vi "derivative.vi"(10 "Starting value":dbl, 11 "x":dbl) -> (3 "dx/dt":dbl)   [LabVIEW 2015]
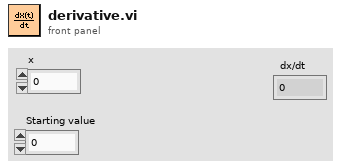
[diagram p1: front panel]
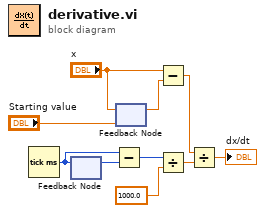
[diagram p0: block diagram]
diagram:
  n1 = Tick Count (ms)() -> (millisecond timer value=w5:u32)
  n2 = feedback #1() -> (w6:u32)  [unwired: 1 in]
  n3 = feedback-in #1(w5) -> ()
  n4 = Subtract(x=w5, y=w6) -> (x-y=w3:u32)
  n5 = feedback #2("Starting value") -> (w10:dbl)
  n6 = feedback-in #2("x") -> ()
  n7 = Subtract(x="x", y=w10) -> (x-y=w8:dbl)
  n8 = Divide(x=w3, y=1000.0) -> (x/y=w1:dbl)
  n9 = Divide(x=w8, y=w1) -> (x/y=→"dx/dt":dbl)
